vi "ROI entry screen-Adjust to correct times.vi"(8 "error in (no error)":errorcluster) -> (0 "error out":errorcluster, 2 "Corrected":bool)   [LabVIEW 2013]
uses:
  Globals/gl_ROI Entry UI globals.vi
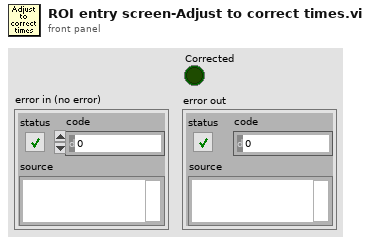
[diagram p1: front panel]
types:
  T1 = enum8{"Enabled", "Disabled", "Disabled and Grayed Out"}
  T2 = typedef "ROI entry screen ctrl refs cluster.ctl" = cluster{"Done button":refnum<vi>, "Imaging button":refnum<vi>, "Acquisition button":refnum<vi>, "POI dwell time (us)":refnum<vi>, "Scan dwell time per pixel (us)":refnum<vi>, "# of planes":refnum<vi>, "Zoom":refnum<vi>, "Equal size":refnum<vi>, "Channel":refnum<vi>, "Image Display":refnum<vi>, "Z-Plane Selector":refnum<vi>, "Number of lines left":refnum<vi>, "Z-stack folder path":refnum<vi>, "POI Density":refnum<vi>, "Arb Plane Entry":refnum<vi>, "Whole plane":refnum<vi>, "Clear Last":refnum<vi>, "Clear All":refnum<vi>, "Trial Length (sec)":refnum<vi>, "Palette Type":refnum<vi>, "Intensity slider":refnum<vi>, "# POI":refnum<vi>, "Max Z Proj":refnum<vi>, "Zplane ind":refnum<vi>, "Wavelength (nm)":refnum<vi>, "Number of Trials":refnum<vi>, "Funct stim.trig.enable":refnum<vi>, "Funct stim.trig.delay (s)":refnum<vi>, "Line Mode":refnum<vi>, "Step size (µm)":refnum<vi>, "ROI move mode":refnum<vi>, "Cool-down time (s)":refnum<vi>, "Enable cool-down time":refnum<vi>, "Motor Z ind. (um)":refnum<vi>, "AOL Z ind. (um)":refnum<vi>}
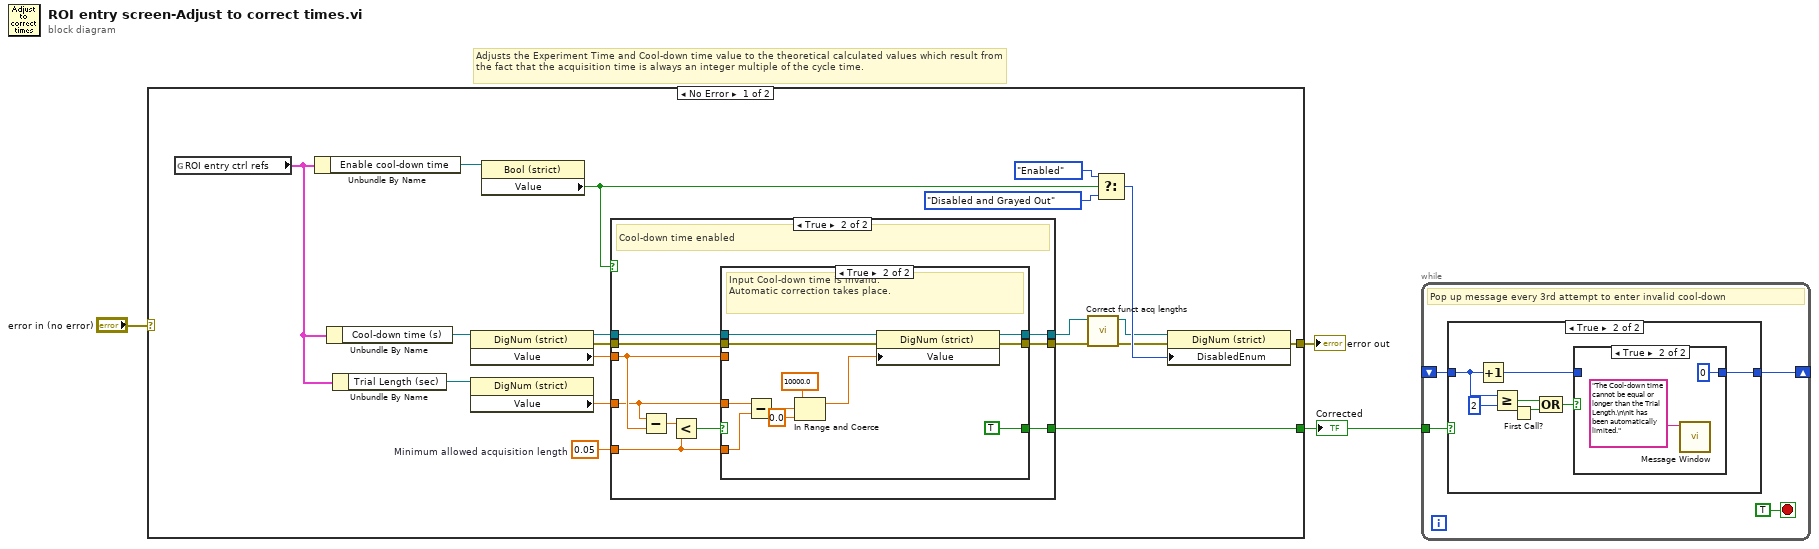
[diagram p0: block diagram]
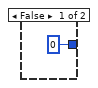
[diagram p2: hidden frame]
diagram:
  # "Adjusts the Experiment Time and Cool-down time value to the theoretical calculated values which result from the fact that the acquisition time is always an integer multiple of the cycle time."
  n1 = case shown="No Error" "error in (no error)" {
    selector: "error in (no error)" -> [_ w48]
    tunnel: [w17 w48] -> w3
    tunnel: [w16 _] -> w1
    frame No Error {
      w7 = 0.05  # Minimum allowed acquisition length
      n2 = global read "gl_ROI Entry UI globals.vi" "ROI entry ctrl refs"() -> (w18:T2)
      n3 = Unbundle By Name(w18) -> ("Enable cool-down time"=w22:refnum<vi>)
      n4 = Unbundle By Name(w18) -> ("Cool-down time (s)"=w21:refnum<vi>)
      n5 = Unbundle By Name(w18) -> ("Trial Length (sec)"=w19:refnum<vi>)
      n6 = property on="Property Node" class="DigNum (strict)"(reference=w21) -> (reference out=w11:refnum<vi>, error out=w10:errorcluster, "Value"=w9:dbl)  [unwired: 1 in]
      n7 = property on="Property Node" class="DigNum (strict)"(reference=w19) -> ("Value"=w8:dbl)  [unwired: 1 in, 2 out]
      n8 = property on="Property Node" class="Bool (strict)"(reference=w22) -> ("Value"=w6:bool)  [unwired: 1 in, 2 out]
      n9 = case shown="True" w6 {
        tunnel: w11 -> [w23 w32]
        tunnel: w10 -> [w24 w31]
        tunnel: w9 -> [_ w30]
        tunnel: [w23 w29] -> w4
        tunnel: [w24 w28] -> w5
        tunnel: w8 -> [_ w27]
        tunnel: w7 -> [_ w26]
        tunnel: [_ w25] -> w16
        frame False {
          # "Cool-down time disabled."
        }
        frame True {
          # "Cool-down time enabled"
          n10 = Subtract(x=w27, y=w30) -> (x-y=w34:dbl)
          n11 = Less?(x=w34, y=w26) -> (x < y?=w33:bool)
          n12 = case shown="True" w33 {
            tunnel: w32 -> [w35 w47]
            tunnel: w31 -> [w36 w46]
            tunnel: w30 -> [_ _]
            tunnel: [w35 w45] -> w29
            tunnel: [w36 w44] -> w28
            tunnel: w27 -> [_ w43]
            tunnel: w26 -> [_ w42]
            tunnel: [_ TRUE] -> w25
            frame False {
              # "Input Cool-down time is valid"
            }
            frame True {
              # "Input Cool-down time is invalid.\nAutomatic correction takes place."
              n13 = Subtract(x=w43, y=w42) -> (x-y=w41:dbl)
              n14 = In Range and Coerce(upper limit=10000.0, x=w41, lower limit=0.0) -> (coerced(x)=w38:dbl)  [unwired: 1 out]
              n15 = property on="Property Node" class="DigNum (strict)"(reference=w47, error in=w46, "Value"=w38) -> (reference out=w45:refnum<vi>, error out=w44:errorcluster)
            }
          }
        }
      }
      n16 = call "Correct funct acq lengths.vi"("error in (no error)"=w5, "Cool-down time (s)"=w4) -> ("error out"=w14:errorcluster, "Cool-down time (s)"=w15:refnum<vi>)  [unwired: 7 in, 1 out]
      n17 = Select(t=T1."Enabled" ("Disabled"), s=w6, f=T1."Disabled and Grayed Out" ("Disabled")) -> (s? t:f=w20:T1)
      n18 = property on="Property Node" class="DigNum (strict)"(reference=w15, error in=w14, "DisabledEnum"=w20) -> (error out=w17:errorcluster)  [unwired: 1 out]
    }
    frame Error {
    }
  }
  "error out" <- w3
  "Corrected" <- w1
  n19 = while {
    shift-right: [w49] -> _
    shift-left: _ -> [w51]
    tunnel: w1 -> [w50]
    stop <- TRUE stop-if-true
    # "Pop up message every 3rd attempt to enter invalid cool-down"
    n20 = case shown="True" w50 {
      tunnel: w51 -> [_ w55]
      tunnel: [0 w56] -> w49
      frame False {
      }
      frame True {
        n21 = Increment(x=w55) -> (x+1=w57:i32)
        n22 = Greater Or Equal?(x=w55, y=2) -> (x >= y?=w58:bool)
        n23 = First Call?() -> (First Call?: T/F=w60:bool)
        n24 = Compound Arithmetic op=OR(w58, w60) -> (w59:bool)
        n25 = case shown="True" w59 {
          tunnel: w57 -> [w61 _]
          tunnel: [w61 0] -> w56
          frame False {
          }
          frame True {
            n26 = call "Message Window.vi"("Message string"="The Cool-down time cannot be equal or longer than the Trial Length.\n\nIt has been automatically limited.") -> ()  [unwired: 10 in, 1 out]
          }
        }
      }
    }
  }
